vi "Scale Waveform.vi"(10 "coefficient info":T1(array[cluster]), 11 "wfm":i16[][](array[numeric])) -> (3 "Array":dbl[][](array[numeric]))   [LabVIEW 2018]
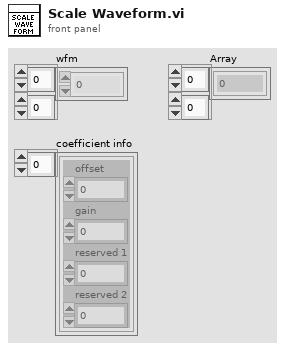
[diagram p1: front panel]
types:
  T1 = cluster{"offset":dbl, "gain":dbl, "reserved 1":dbl, "reserved 2":dbl}[]
  T2 = cluster{"offset":dbl, "gain":dbl, "reserved 1":dbl, "reserved 2":dbl}
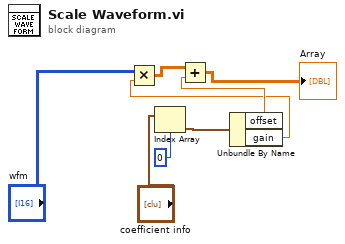
[diagram p0: block diagram]
diagram:
  n1 = Index Array(array="coefficient info", index=0) -> (element=w4:T2)
  n2 = Unbundle By Name(w4) -> ("offset"=w7:dbl, "gain"=w5:dbl)
  n3 = Multiply(x="wfm", y=w5) -> (x*y=w6:dbl[][])
  n4 = Add(x=w6, y=w7) -> (x+y=→"Array":dbl[][])
